vi "NEMA Unbalance.vi"(0 "voltage RMS values":dbl[](array[numeric]), 11 "error in (no error)":errorcluster) -> (4 "unbalance [%]":dbl[](array[numeric]), 6 "unbalance derating factors":dbl[](array[numeric]) format="%#_3f", 15 "error out":errorcluster)   [LabVIEW 2014, in "NI_EP_Motor Monitoring.lvlib"]
doc: "Calculates the unbalance in compliance with NEMA MG 1-2014."
uses:
  <vilib>/addons/Electrical Power/Motor Monitoring/NI_EP_Motor Monitoring.lvlib
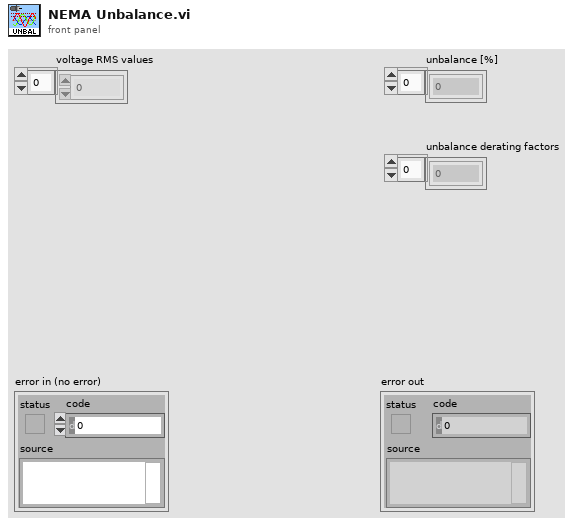
[diagram p1: front panel]
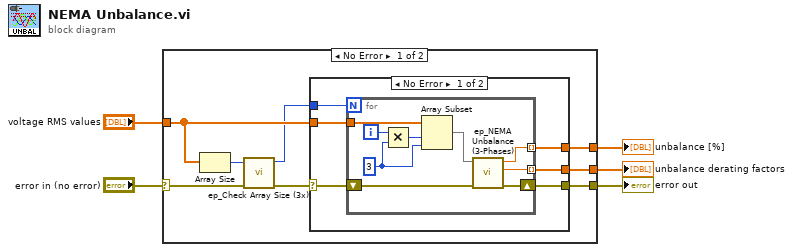
[diagram p0: block diagram]
diagram:
  n1 = case shown="No Error" "error in (no error)" {
    selector: "error in (no error)" -> [w10 w30]
    tunnel: "voltage RMS values" -> [w8 _]
    tunnel: [w13 _] -> w5
    tunnel: [w12 _] -> w4
    tunnel: [w11 w30] -> w3
    frame No Error {
      n2 = Array Size(array=w8) -> (size(s)=w9:i32)
      n3 = call <vilib>:"ep_Check Array Size (3x).vi"("error in (no error)"=w10, "number of channels"=w9) -> ("error out"=w6:errorcluster, "number of 3 phases"=w7:i32)  [unwired: 8 in]
      n4 = case shown="No Error" w6 {
        selector: w6 -> [w14 w29]
        tunnel: [w19 _] -> w13
        tunnel: [w18 _] -> w12
        tunnel: [w17 w29] -> w11
        tunnel: w8 -> [w16 _]
        tunnel: w7 -> [w15 _]
        frame No Error {
          n5 = for {
            N: w15 -> [_]
            tunnel: [w28] -> w19 mode=indexing
            tunnel: [w27] -> w18 mode=indexing
            shift-right: [w25] -> w17
            shift-left: w14 -> [w26]
            tunnel: w16 -> [w21]
            i -> [w24]
            w23 = 3 ("dimension size")
            n6 = Multiply(x=w24, y=w23) -> (x*y=w22:i32)
            n7 = Array Subset(array=w21, index=w22, length=w23) -> (w20:dbl[])
            n8 = call <vilib>:"ep_NEMA Unbalance (3-Phases).vi"("error in (no error)"=w26, "voltage RMS values (3-phases)"=w20) -> ("error out"=w25:errorcluster, "unbalance derating factor"=w27:dbl, "unbalance [%]"=w28:dbl)  [unwired: 7 in]
          }
        }
        frame Error {
        }
      }
    }
    frame Error {
    }
  }
  "error out" <- w3
  "unbalance derating factors" <- w4
  "unbalance [%]" <- w5
